vi "Convert Wheel Counts to Position.vi"(7 "Count Tollerance":i32=3, 10 "PPR":i32=1024, 11 "Wheel Count":i32) -> (3 "Current Positions Out":T1)   [LabVIEW 2023, in "Tube Wheel_ACT.lvlib"]
uses:
  Tube Wheel_ACT.lvlib
  Shared Code/TypeDefs/ENUM_Tube Wheel Positions.ctl
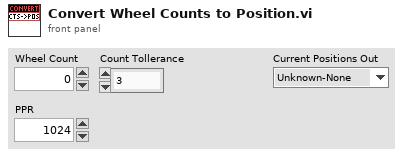
[diagram p1: front panel]
types:
  T1 = typedef "ENUM_Tube Wheel Positions.ctl" = enum16{"Unknown-None", "Tube Red A", "Tube Black B", "Tube Red C", "Tube Black D", "Tube Red E", "Tube Black F", "Load A-B", "Load B-C", "Load C-D", "Load D-E", "Load E-F", "Load F-A"}
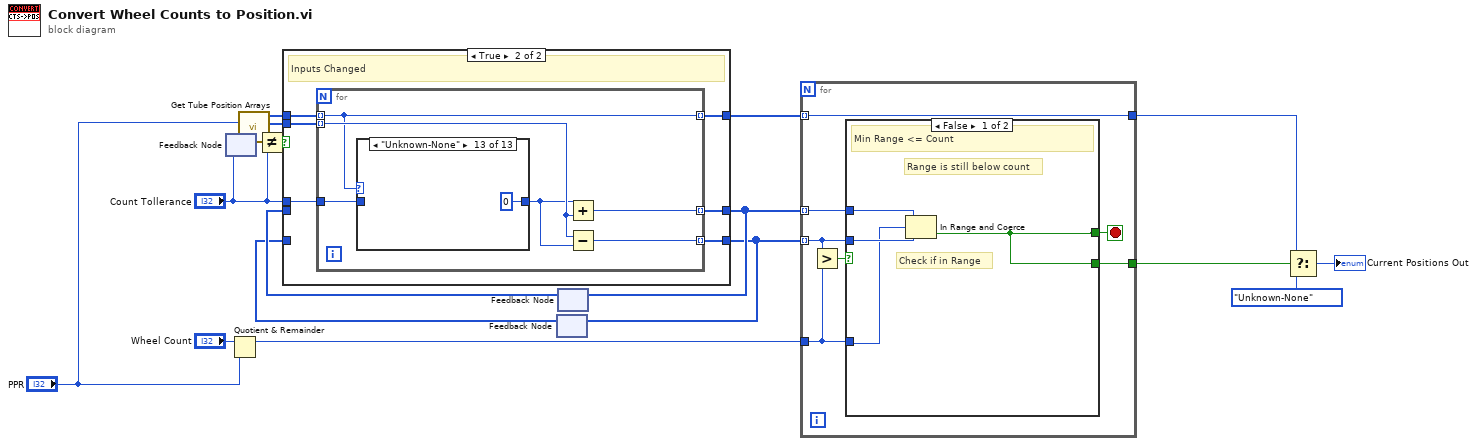
[diagram p0: block diagram]
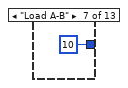
[diagram p9: hidden frame]
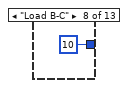
[diagram p10: hidden frame]
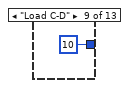
[diagram p11: hidden frame]
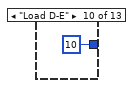
[diagram p12: hidden frame]
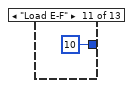
[diagram p13: hidden frame]
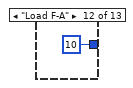
[diagram p14: hidden frame]
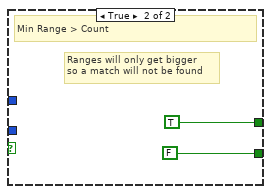
[diagram p15: hidden frame]
diagram:
  n1 = feedback #1() -> (w11:i32)  [unwired: 1 in]
  n2 = feedback-in #1("Count Tollerance") -> ()
  n3 = Quotient & Remainder(x="Wheel Count", y="PPR") -> (x-y*floor(x/y)=w16:i32)  [unwired: 1 out]
  n4 = call "Get Tube Position Arrays.vi"("PPR"="PPR") -> ("Counts"=w3:i32[], "Positons"=w4:T1[])  [unwired: 9 in]
  n5 = Not Equal?(x=w11, y="Count Tollerance") -> (x != y?=w2:bool)
  n6 = feedback #2() -> (w6:i32[])  [unwired: 1 in]
  n7 = feedback #3() -> (w7:i32[])  [unwired: 1 in]
  n8 = case shown="True" w2 {
    tunnel: w3 -> [_ w23]
    tunnel: w4 -> [w18 w22]
    tunnel: [w18 w21] -> w5
    tunnel: "Count Tollerance" -> [_ w24]
    tunnel: [w19 w26] -> w8
    tunnel: [w20 w25] -> w9
    tunnel: w7 -> [w20 _]
    tunnel: w6 -> [w19 _]
    frame False {
      # "Inputs are the Same"
    }
    frame True {
      # "Inputs Changed"
      n9 = for {
        tunnel: [w32] -> w26 mode=indexing
        tunnel: [w31] -> w25 mode=indexing
        tunnel: w24 -> [w29]
        tunnel: w23 -> [w30] mode=indexing
        tunnel: w22 -> [w27] mode=indexing
        tunnel: [w27] -> w21 mode=indexing
        n10 = case shown="\"Unknown-None\"" w27 {
          tunnel: w29 -> [w33 w34 w35 w36 w37 w38 _ _ _ _ _ _ _]
          tunnel: [w33 w34 w35 w36 w37 w38 10 ("Count Tollerance") 10 ("Count Tollerance") 10 ("Count Tollerance") 10 ("Count Tollerance") 10 ("Count Tollerance") 10 ("Count Tollerance") 0 ("Count Tollerance")] -> w28
          frame "Tube Red A" {
          }
          frame "Tube Black B" {
          }
          frame "Tube Red C" {
          }
          frame "Tube Black D" {
          }
          frame "Tube Red E" {
          }
          frame "Tube Black F" {
          }
          frame "Load A-B" {
          }
          frame "Load B-C" {
          }
          frame "Load C-D" {
          }
          frame "Load D-E" {
          }
          frame "Load E-F" {
          }
          frame "Load F-A" {
          }
          frame "Unknown-None" {
          }
        }
        n11 = Add(x=w28, y=w30) -> (x+y=w31:i32)
        n12 = Subtract(x=w30, y=w28) -> (x-y=w32:i32)
      }
    }
  }
  n13 = feedback-in #2(w8) -> ()
  n14 = feedback-in #3(w9) -> ()
  n15 = for {
    tunnel: w16 -> [w46]
    tunnel: w5 -> [w52] mode=indexing
    tunnel: w9 -> [w47] mode=indexing
    tunnel: w8 -> [w51] mode=indexing
    tunnel: [w52] -> w14
    tunnel: [w48] -> w15
    stop <- w49 stop-if-true
    n16 = Greater?(x=w51, y=w46) -> (0:w50:bool)
    n17 = case shown="False" w50 {
      tunnel: w51 -> [w55 _]
      tunnel: [w53 TRUE] -> w49
      tunnel: [w53 FALSE] -> w48
      tunnel: w47 -> [w56 _]
      tunnel: w46 -> [w54 _]
      frame False {
        # "Check if in Range"
        # "Range is still below count"
        # "Min Range <= Count"
        n18 = In Range and Coerce(upper limit=w56, x=w54, lower limit=w55) -> (In Range?=w53:bool)  [unwired: 1 out]
      }
      frame True {
        # "Ranges will only get bigger\nso a match will not be found"
        # "Min Range > Count"
      }
    }
  }
  n19 = Select(t=w14, s=w15, f=ENUM_Tube_Wheel_Positions."Unknown-None") -> (s? t:f=→"Current Positions Out":T1)
